vi "CleanTxtFile.vi"   [LabVIEW 2020]
panel:
  # "This VI write \"Sample Text\" string to a txt file, \nthen clearn the contents by setting the file size to 0."
types:
  T1 = enum16{"open", "replace", "create", "open or create", "replace or create", "replace or create with confirmation"}
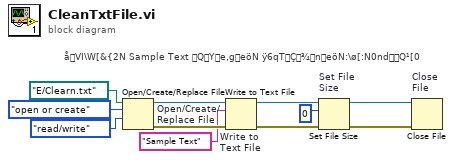
[diagram p0: block diagram]
diagram:
  # "åVI\\W[&{2N Sample Text QYe,geöN ÿ6qTÇ¾neöN:\\ø[:N0ndQ¹[0"
  n1 = Open/Create/Replace File "Open/Create/\nReplace File"(file path (use dialog)=path "E:/Clearn.txt", operation (0:open)=T1."open or create", access (0:read/write)=enum16{"read/write", "read-only", "write-only"}."read/write") -> (refnum out=w5:refnum<file>, error out=w4:errorcluster)  [unwired: 3 in, 1 out]
  n2 = Write to Text File "Write to\nText File"(file (use dialog)=w5, text="Sample Text", error in=w4) -> (refnum out=w6:refnum<file>, error out=w3:errorcluster)  [unwired: 1 in, 1 out]
  n3 = Set File Size "Set File\nSize"(4:w3, 6:i64 0 ("size (in bytes)"), 7:w6) -> (0:w8:errorcluster, 3:w7:refnum<file>)
  n4 = Close File "Close\nFile"(refnum=w7, error in=w8) -> ()  [unwired: 2 out]
